vi "Cleanup Error String.vi"(8 "error in (no error)":errorcluster) -> (0 "error out":errorcluster)   [LabVIEW 2024, in "StreamWriter.lvlib" / "StreamWriter.lvclass"]
uses:
  StreamWriter.lvclass
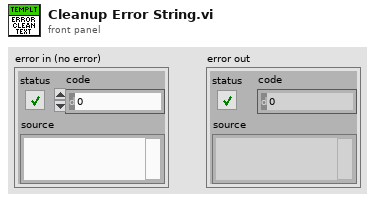
[diagram p1: front panel]
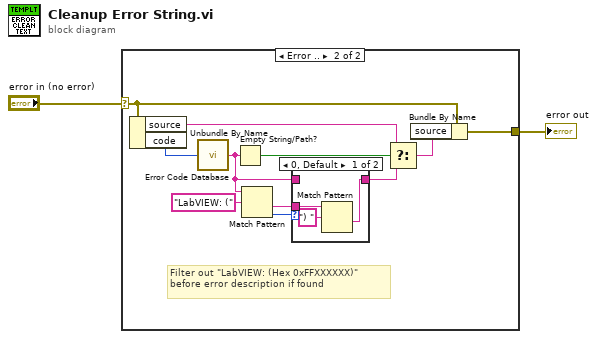
[diagram p0: block diagram]
diagram:
  n1 = case shown="Error .." "error in (no error)" {
    selector: "error in (no error)" -> [w3 w13]
    tunnel: [w3 w9] -> w1
    frame No Error {
    }
    frame Error {
      # "Filter out \"LabVIEW: (Hex 0xFFXXXXXX)\" before error description if found"
      n2 = Unbundle By Name(w13) -> ("source"=w11:string, "code"=w14:i32)
      n3 = call <vilib>:"Error Code Database.vi"("Error Code"=w14) -> ("Error Text"=w5:string)
      n4 = Empty String/Path?(string/path=w5) -> (empty?=w12:bool)
      n5 = Match Pattern(string=w5, regular expression="LabVIEW: (") -> (after substring=w6:string, offset past match=w7:i32)  [unwired: 1 in, 2 out]
      n6 = case shown="0, Default" w7 {
        tunnel: w6 -> [w17 _]
        tunnel: w5 -> [_ w18]
        tunnel: [w15 w18] -> w4
        frame 0, Default {
          n7 = Match Pattern(string=w17, regular expression=") ") -> (after substring=w15:string)  [unwired: 1 in, 3 out]
        }
        frame -1 {
        }
      }
      n8 = Select(t=w11, s=w12, f=w4) -> (s? t:f=w10:string)
      n9 = Bundle By Name(cluster=w13, "source"=w10) -> (w9:errorcluster)
    }
  }
  "error out" <- w1
